vi "UI_set velocity.vi"(8 "error in (no error)":errorcluster, 10 "device index":T2, 11 "velocity set":T1) -> (0 "error out":errorcluster, 1 "旋转电机速度":dbl, 2 "平移电机速度":dbl)   [LabVIEW 2017]
uses:
  device control/device index.ctl
  velocity set control.ctl
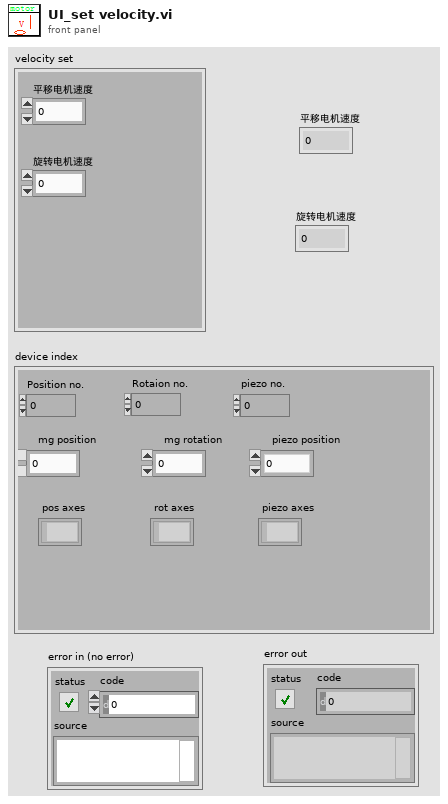
[diagram p1: front panel]
types:
  T1 = typedef "velocity set control.ctl" = cluster{"平移电机速度":dbl, "旋转电机速度":dbl}
  T2 = typedef "device index.ctl" = cluster{"Position no.":i32, "Rotaion no.":i32, "piezo no.":i32, "mg position":dbl, "mg rotation":dbl, "piezo position":dbl, "pos axes":string[], "rot axes":string[], "piezo axes":string[]}
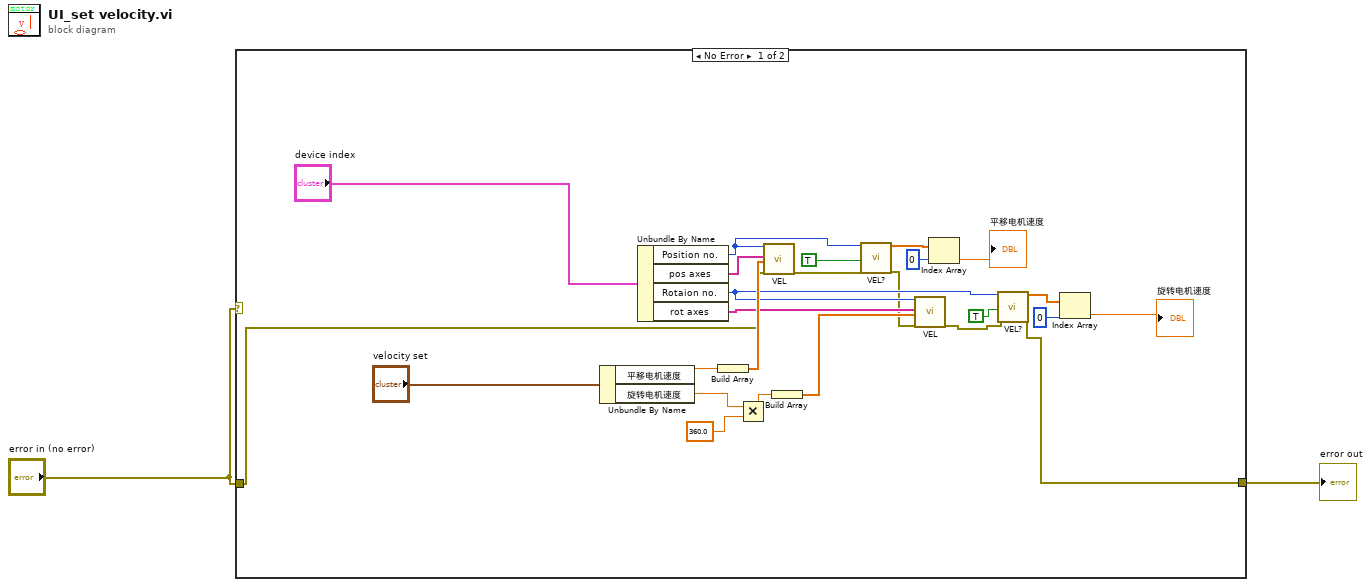
[diagram p0: block diagram]
diagram:
  n1 = case shown="No Error" "error in (no error)" {
    tunnel: "error in (no error)" -> [w5 w28]
    tunnel: [w3 w28] -> w1
    frame No Error {
      n2 = Unbundle By Name("velocity set") -> ("平移电机速度"=w19:dbl, "旋转电机速度"=w9:dbl)
      n3 = Unbundle By Name("device index") -> ("Position no."=w16:i32, "pos axes"=w17:string[], "Rotaion no."=w18:i32, "rot axes"=w6:string[])
      n4 = Build Array(w19) -> (w20:dbl[])
      n5 = Multiply(x=w9, y=360.0) -> (x*y=w7:dbl)
      n6 = call "VEL.vi"("System no."=w16, "Axes to set"=w17, "Velocity values"=w20, "error in"=w5) -> ("error out"=w15:errorcluster)  [unwired: 14 in, 1 out]
      n7 = Build Array(w7) -> (w21:dbl[])
      n8 = call "VEL?.vi"("System no."=w16, "All axes?"=TRUE, "error in"=w15) -> ("Velocity"=w23:dbl[], "error out"=w4:errorcluster)  [unwired: 15 in]
      n9 = call "VEL.vi"("System no."=w18, "Axes to set"=w6, "Velocity values"=w21, "error in"=w4) -> ("error out"=w14:errorcluster)  [unwired: 14 in, 1 out]
      n10 = Index Array(array=w23, index=0 ("索引")) -> (element=→"平移电机速度":dbl)
      n11 = call "VEL?.vi"("System no."=w18, "All axes?"=TRUE, "error in"=w14) -> ("Velocity"=w25:dbl[], "error out"=w3:errorcluster)  [unwired: 15 in]
      n12 = Index Array(array=w25, index=0 ("索引")) -> (element=→"旋转电机速度":dbl)
    }
    frame Error {
    }
  }
  "error out" <- w1
